vi "SetDisplayItems__slk_mt.vi"(8 "error in (no error)":errorcluster, 11 "tree view in":refnum<class "TreeView__slk_mt.lvclass">) -> (0 "error out":errorcluster, 3 "tree view out":refnum<class "TreeView__slk_mt.lvclass">)   [LabVIEW 2014, in "Lazyboots Menu Tool.lvlib" / "TreeView__slk_mt.lvclass"]
doc: "Sets display items and theirs open status."
uses:
  TreeView__slk_mt.lvclass
  TreeView__slk_mt.lvclass/TreeView__slk_mt.ctl
panel:
  # "SetDisplayItems__slk_mt.vi\nSets display items and theirs open status.\n\nNOTICE -- YOU MUST LEAVE THIS NOTICE IN PLACE.\n\nCopyright (c) 2011, LIANG LIU Shawn.Liu.cn@gmail.com\nAll rights reserved.\n\nRedistribution and use in source and binary forms, with or without modification, are permitted provided that the following conditions are met:\n-Redistributions of source code must retain the above copyright notice, this list of conditions and the following disclaimer.\n-Redistributions in binary form must reproduce the above copyright notice, this list of conditions and the following disclaimer in the documentation and/or other materials provided with the distribution.\n-Neither the name of the eLp nor the names of its contributors may be used to endorse or promote products derived from this software without specific prior written permission.\n\nTHIS SOFTWARE IS PROVIDED BY THE COPYRIGHT HOLDERS AND CONTRIBUTORS \"AS IS\" AND ANY EXPRESS OR IMPLIED WARRANTIES, INCLUDING, BUT NOT LIMITED TO, THE IMPLIED WARRANTIES OF MERCHANTABILITY AND FITNESS FOR A PARTICULAR PURPOSE ARE DISCLAIMED. IN NO EVENT SHALL THE COPYRIGHT HOLDER OR CONTRIBUTORS BE LIABLE FOR ANY DIRECT, INDIRECT, INCIDENTAL, SPECIAL, EXEMPLARY, OR CONSEQUENTIAL DAMAGES (INCLUDING, BUT NOT LIMITED TO, PROCUREMENT OF SUBSTITUTE GOODS OR SERVICES; LOSS OF USE, DATA, OR PROFITS; OR BUSINESS INTERRUPTION) HOWEVER CAUSED AND ON ANY THEORY OF LIABILITY, WHETHER IN CONTRACT, STRICT LIABILITY, OR TORT (INCLUDING NEGLIGENCE OR OTHERWISE) ARISING IN ANY WAY OUT OF THE USE OF THIS SOFTWARE, EVEN IF ADVISED OF THE POSSIBILITY OF SUCH DAMAGE."
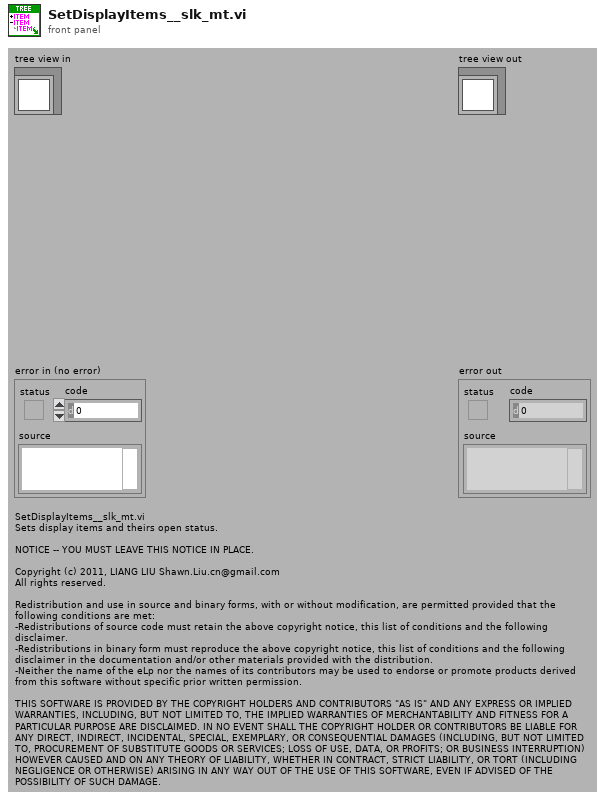
[diagram p1: front panel]
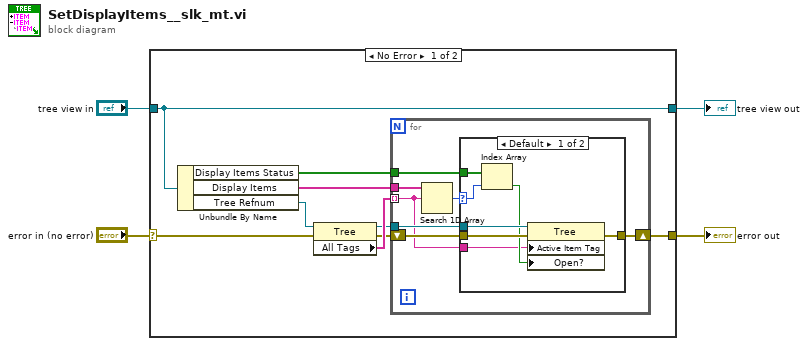
[diagram p0: block diagram]
diagram:
  n1 = case shown="No Error" "error in (no error)" {
    selector: "error in (no error)" -> [w6 w30]
    tunnel: [w5 w30] -> w3
    tunnel: [w13 w29] -> w1
    tunnel: "tree view in" -> [w13 w29]
    frame No Error {
      n2 = Unbundle By Name(w13) -> ("Display Items Status"=w7:bool[], "Display Items"=w12:string[], "Tree Refnum"=w10:refnum<vi>)
      n3 = property class="Tree"(reference=w10, error in=w6) -> (reference out=w9:refnum<vi>, error out=w8:errorcluster, "All Tags"=w11:string[])
      n4 = for {
        tunnel: w12 -> [w20]
        tunnel: w11 -> [w14] mode=indexing
        tunnel: w9 -> [w15]
        shift-right: [w17] -> w5
        shift-left: w8 -> [w18]
        tunnel: w7 -> [w16]
        n5 = Search 1D Array(1D array=w20, element=w14) -> (index of element=w19:i32)  [unwired: 1 in]
        n6 = case shown="Default" w19 {
          selector: w19 -> [w26 _]
          tunnel: w18 -> [w25 w28]
          tunnel: [w23 w28] -> w17
          tunnel: w16 -> [w27 _]
          tunnel: w15 -> [w24 _]
          tunnel: w14 -> [w21 _]
          frame Default {
            n7 = Index Array(array=w27, index=w26) -> (element=w22:bool)
            n8 = property class="Tree"(reference=w24, error in=w25, "Active Item Tag"=w21, "Open?"=w22) -> (error out=w23:errorcluster)  [unwired: 1 out]
          }
          frame -1 {
          }
        }
      }
    }
    frame Error {
    }
  }
  "error out" <- w3
  "tree view out" <- w1
